vi "RFmx_MeasTest_Config.vi"(7 "Meas_Type":string[](array[string])=["ACP"], 8 "error in (no error)":errorcluster, 11 "Instrument Handle in":refnum<k21>="VST") -> (0 "error out":errorcluster, 3 "Instrument Handle out":refnum<k21>="VST")   [LabVIEW 2014]
uses:
  <vilib>/RFmx/RFInstr/mx/RFmxInstr.llb/RFmxInstr Build Signal String.vi
  <vilib>/RFmx/SpecAn/mx/RFmxSpecAn.llb/RFmxSpecAn Select Measurement (Single).vi
panel:
  in  "Reference Level (dBm)":dbl=-15.0 format="%.2f"
  in  "Enable All Traces":bool=TRUE
  in  "IBW (hz)":dbl=3840000.0 format="%.3p"
  in  "Center Freq (Hz)":dbl=1150000000.0 format="%.3p"
  in  "RBW Filter Type":i32(ring)=1 items=["FFT Based", "Gaussian", "Flat", "Synch Tuned - 4", "Synch Tuned - 5"]
  in  "RBW (Hz)":dbl=10000.0 format="%.3p"
  in  "Span (Hz)":dbl=20000000.0 format="%.3p"
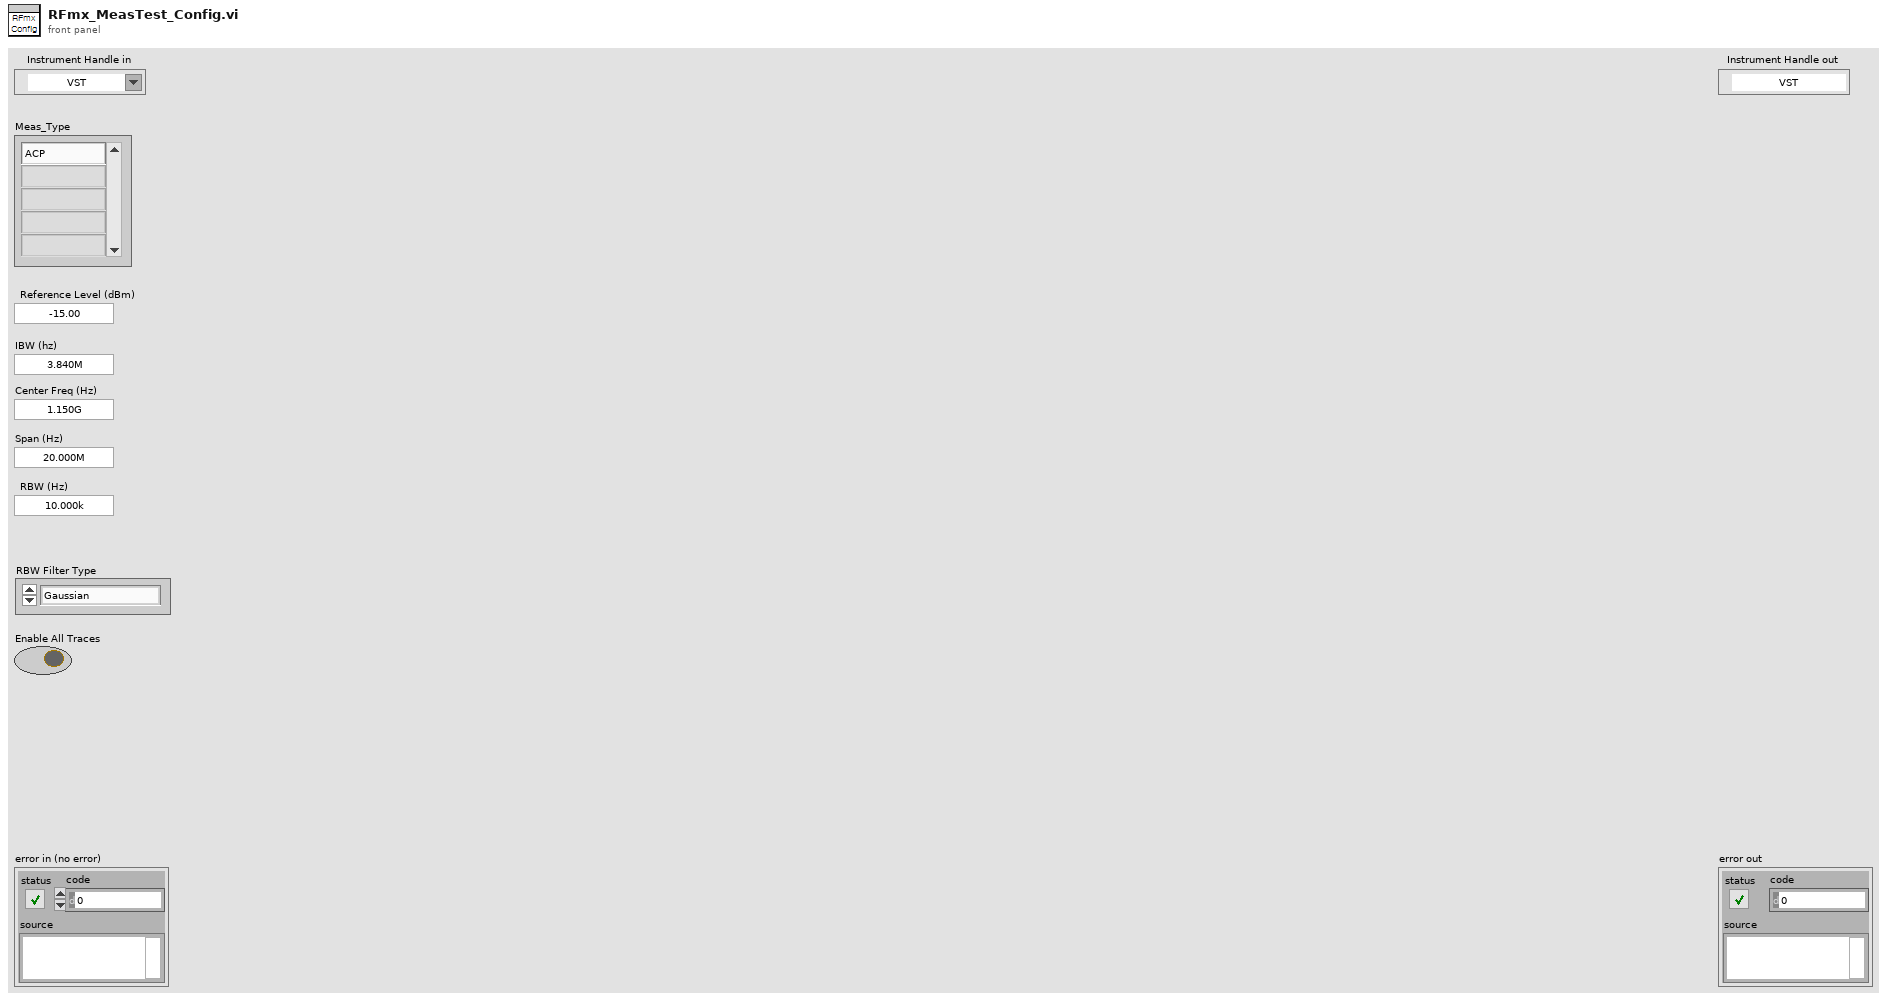
[diagram p1: front panel]
types:
  T1 = enum16{"ACP", "CCDF", "CHP", "FCnt", "Harmonics", "OBW", "SEM", "Spectrum", "Spur", "TXP", "AMPM", "DPD", "IQ"}
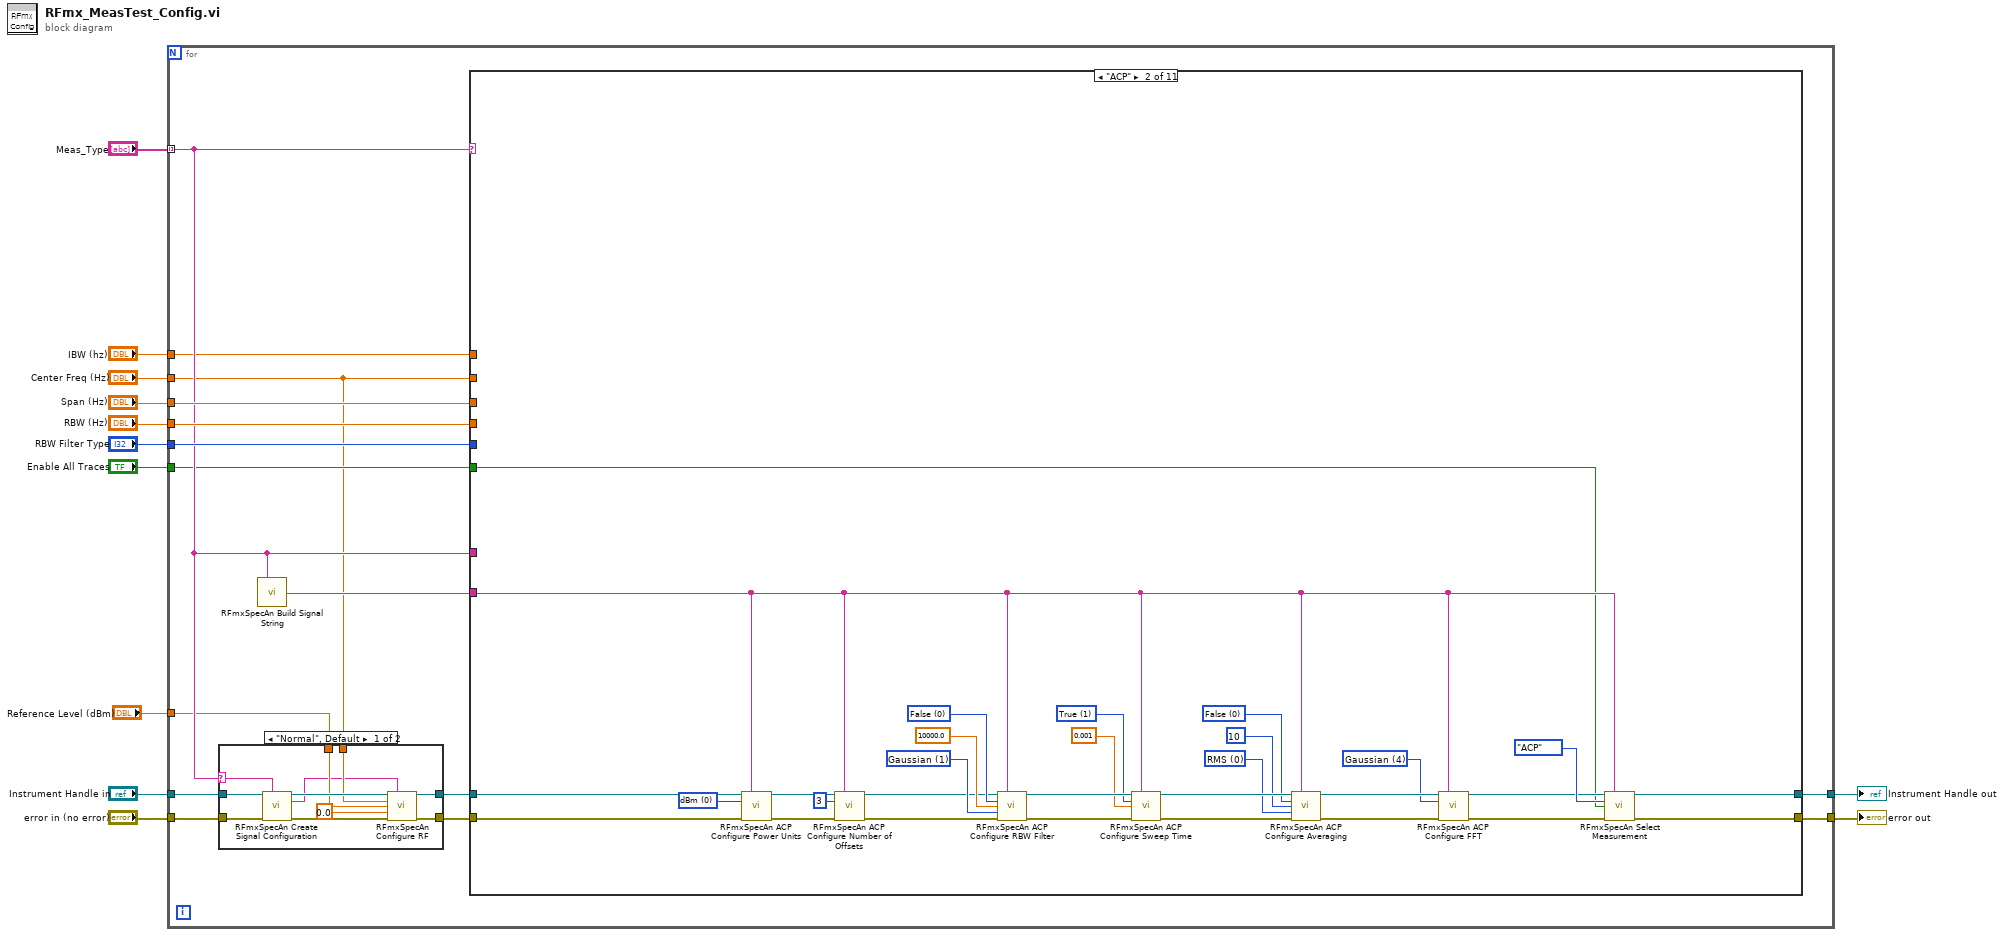
[diagram p0: block diagram]
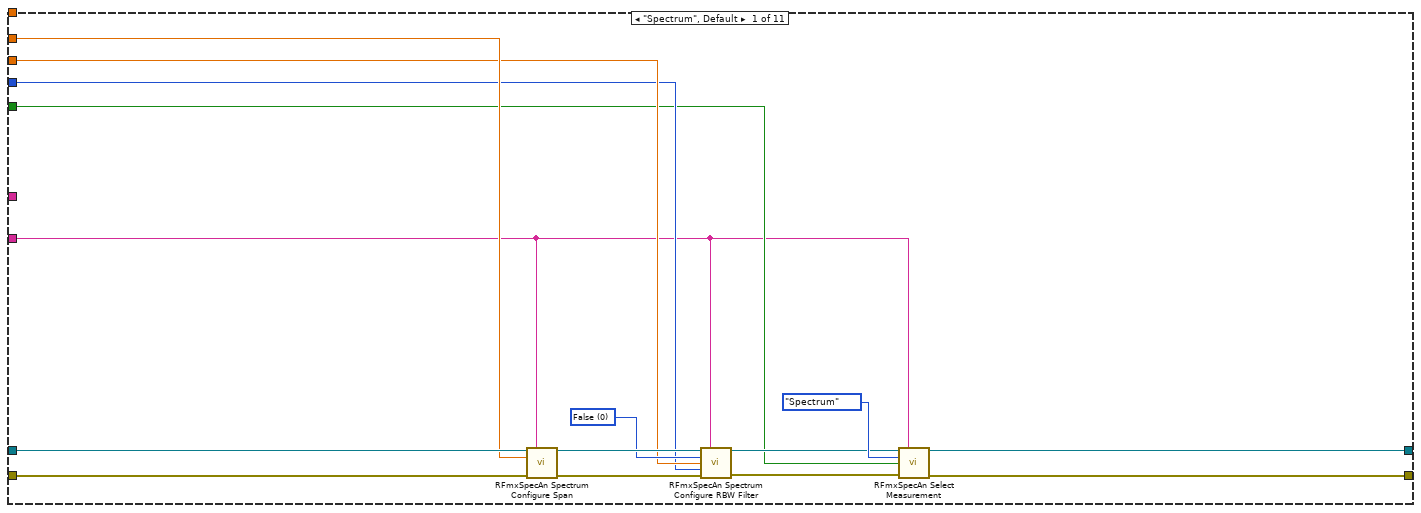
[diagram p3: hidden frame]
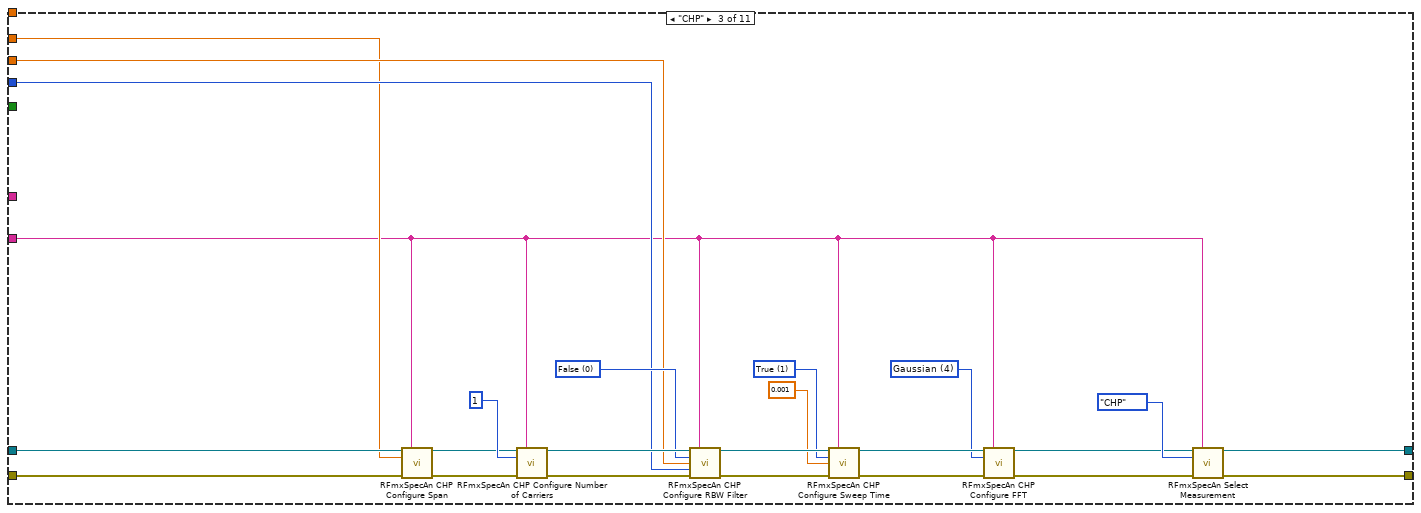
[diagram p4: hidden frame]
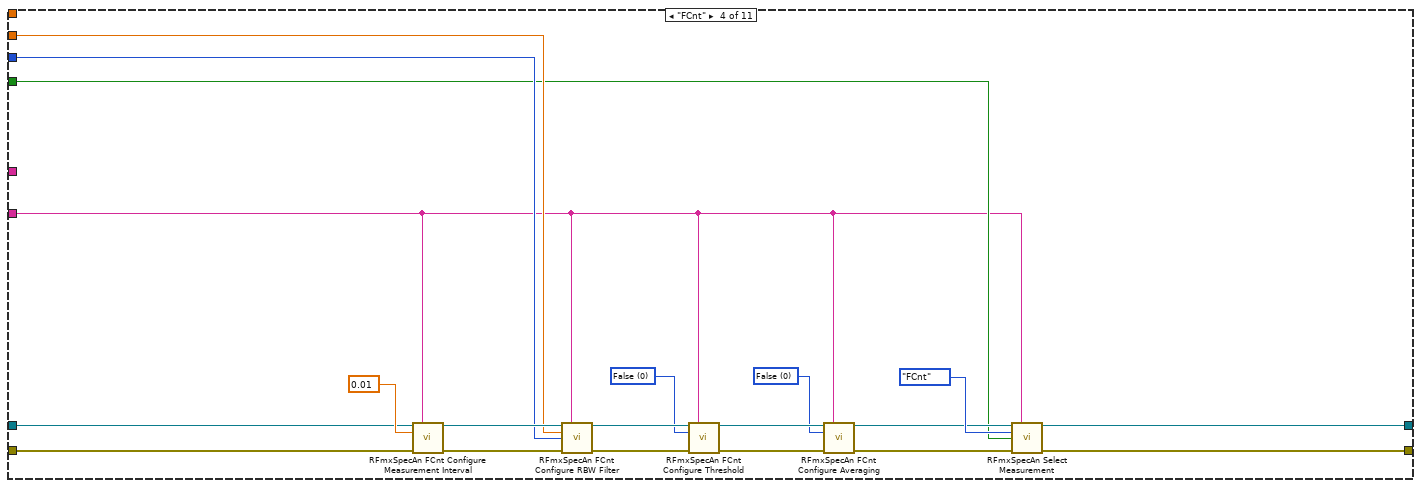
[diagram p5: hidden frame]
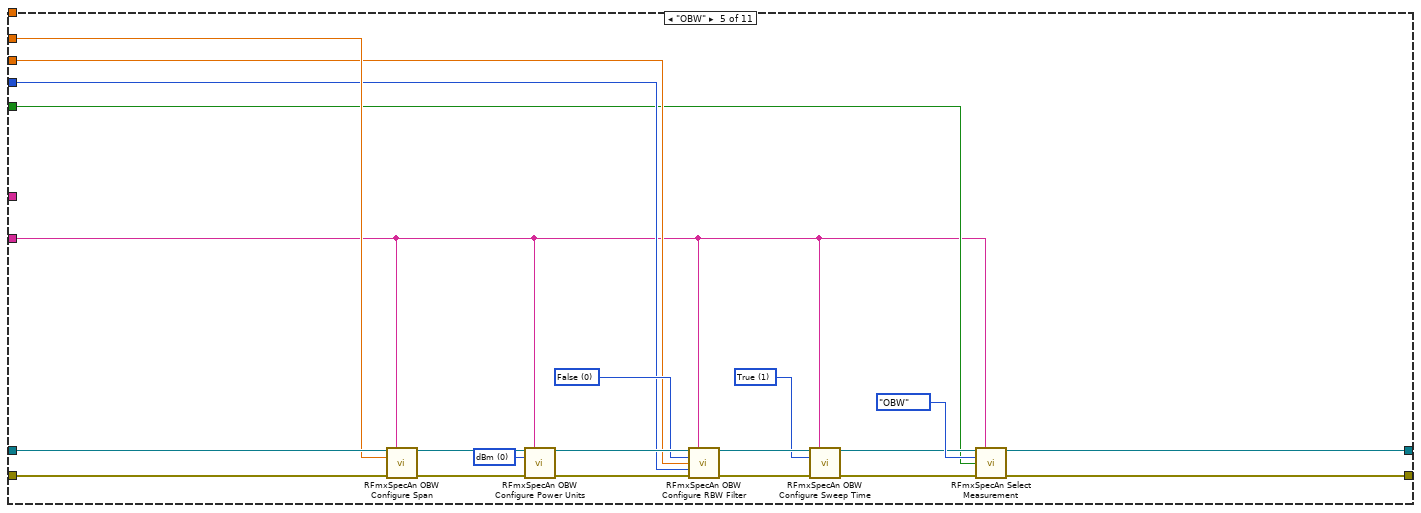
[diagram p6: hidden frame]
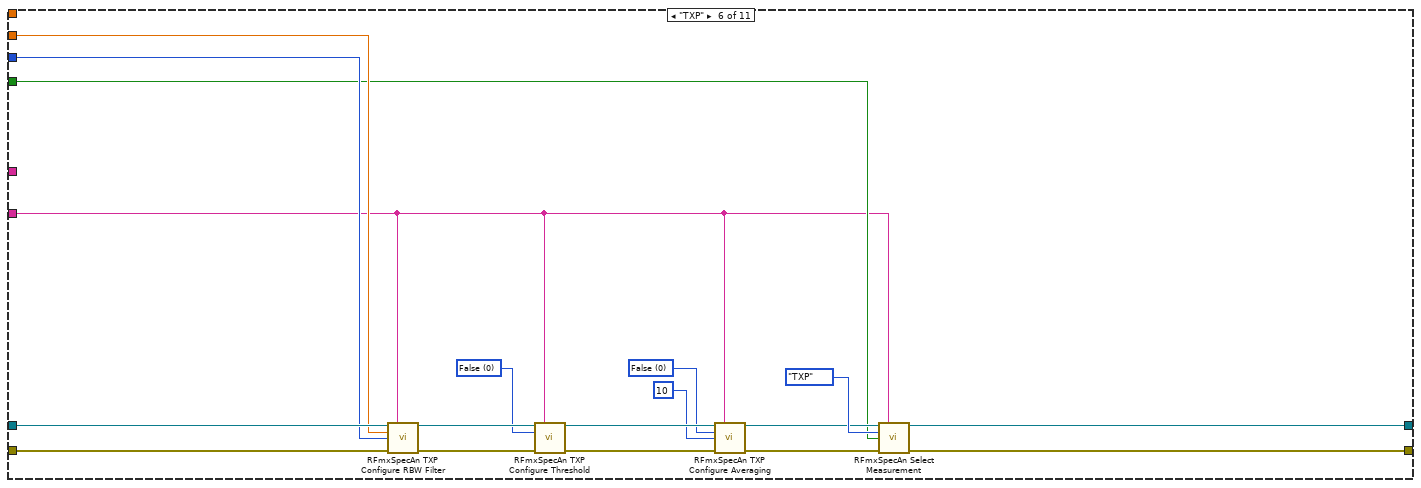
[diagram p7: hidden frame]
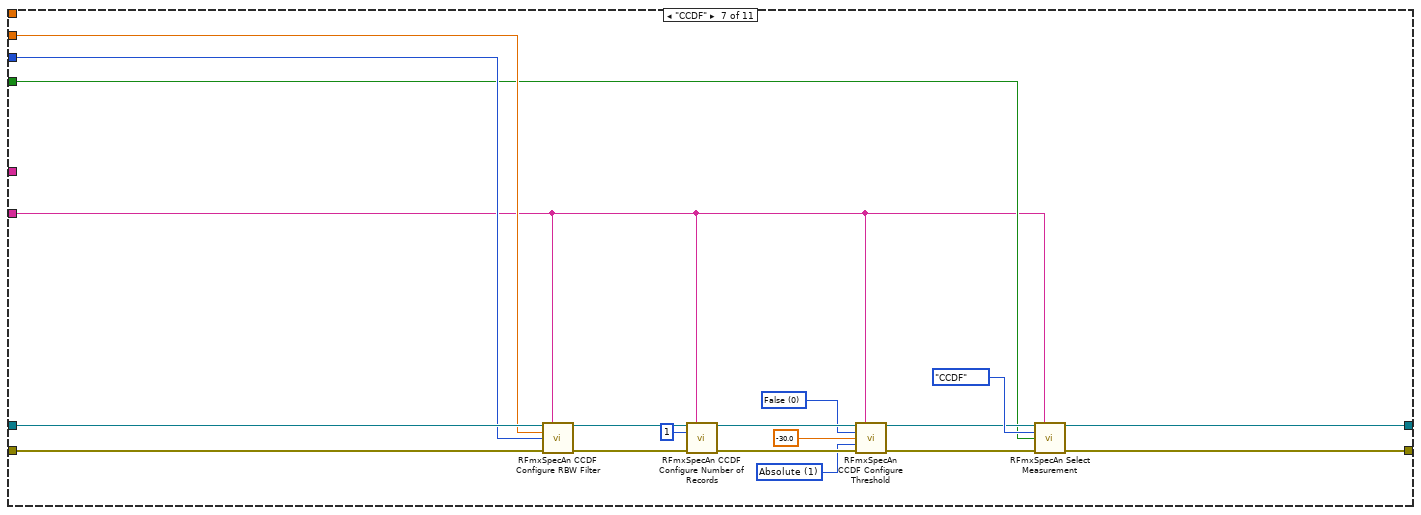
[diagram p8: hidden frame]
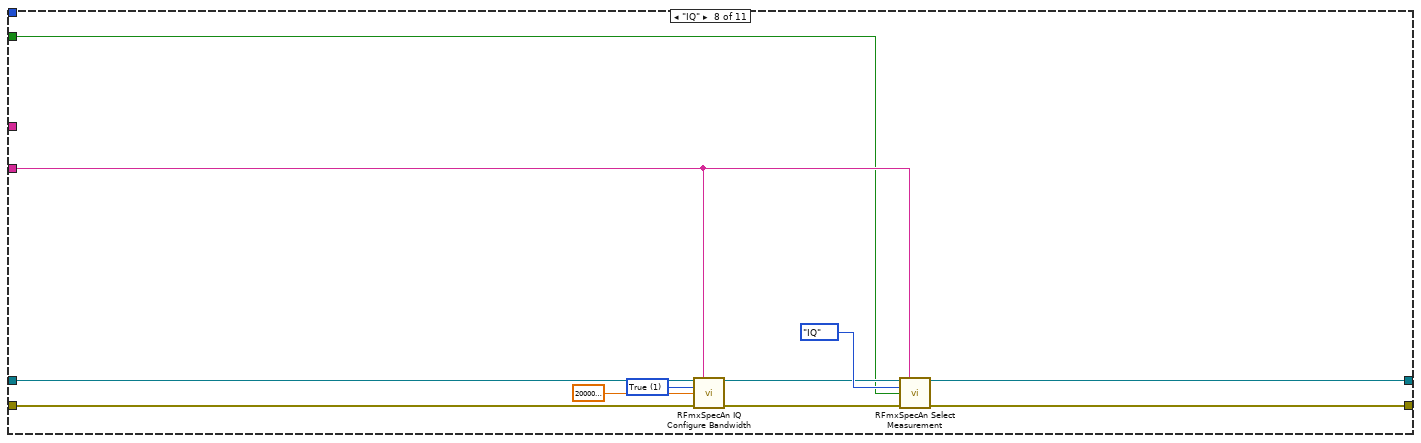
[diagram p9: hidden frame]
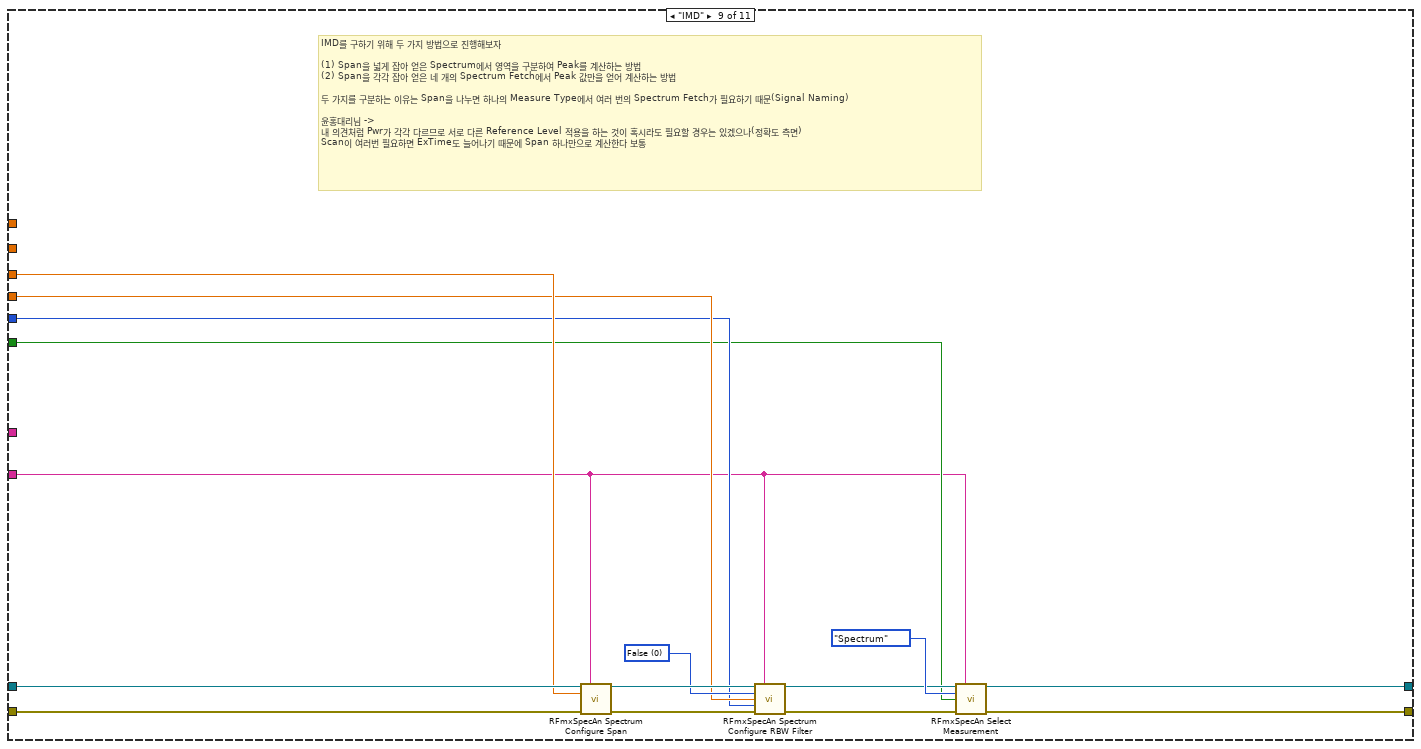
[diagram p10: hidden frame]
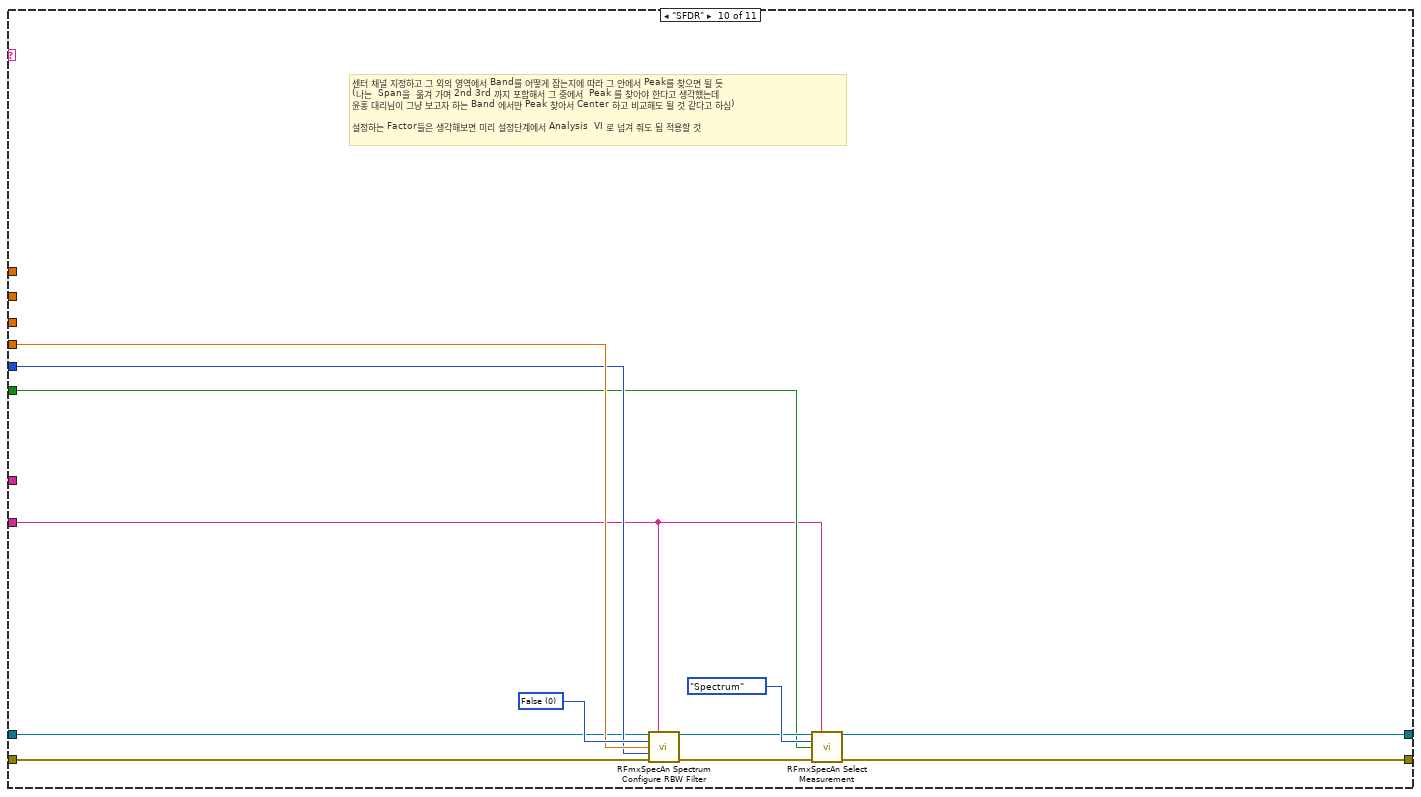
[diagram p11: hidden frame]
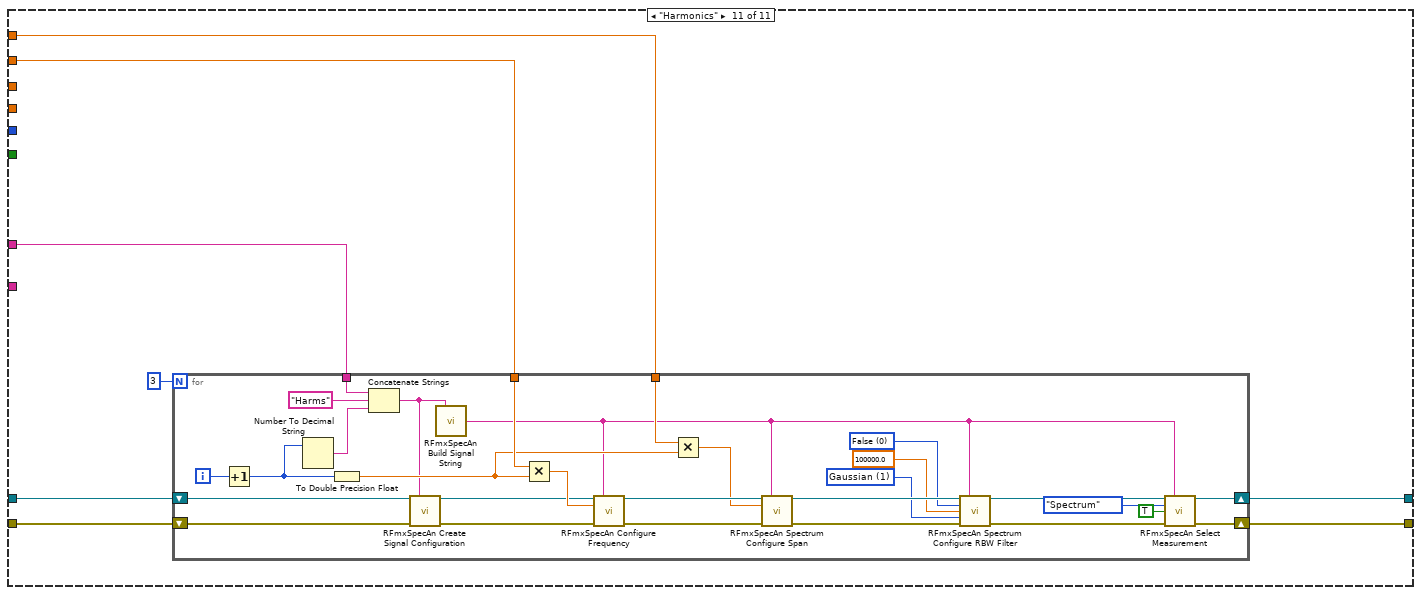
[diagram p12: hidden frame]
diagram:
  n1 = for {
    tunnel: [w27] -> w12
    tunnel: [w26] -> w11
    tunnel: "Meas_Type" -> [w20] mode=indexing
    tunnel: "Instrument Handle in" -> [w22]
    tunnel: "error in (no error)" -> [w21]
    tunnel: "Span (Hz)" -> [w25]
    tunnel: "RBW (Hz)" -> [w24]
    tunnel: "RBW Filter Type" -> [w23]
    tunnel: "Center Freq (Hz)" -> [w15]
    tunnel: "IBW (hz)" -> [w19]
    tunnel: "Enable All Traces" -> [w18]
    tunnel: "Reference Level (dBm)" -> [w16]
    n2 = case shown="\"Normal\", Default" w20 {
      selector: w20 -> [w29 _]
      tunnel: w22 -> [w38 w40]
      tunnel: w21 -> [w37 w39]
      tunnel: [w34 w40] -> w14
      tunnel: [w33 w39] -> w13
      tunnel: w16 -> [w31 _]
      tunnel: w15 -> [w30 _]
      frame "Normal", Default {
        n3 = call <vilib>:"RFmxSpecAn Create Signal Configuration.vi"("Instrument Handle In"=w38, "Signal Name"=w29, "error in (no error)"=w37) -> ("Instrument Handle Out"=w35:refnum<k21>, "Selector String Out"=w28:string, "error out"=w32:errorcluster)  [unwired: 10 in]
        n4 = call <vilib>:"RFmxSpecAn Configure RF.vi"("Instrument Handle In"=w35, "Selector String"=w28, "Center Frequency (Hz)"=w30, "Reference Level (dBm)"=w31, "External Attenuation (dB)"=0.0, "error in (no error)"=w32) -> ("Instrument Handle Out"=w34:refnum<k21>, "error out"=w33:errorcluster)  [unwired: 8 in]
      }
      frame "Harmonics" {
      }
    }
    n5 = call <vilib>:"RFmxSpecAn Build Signal String.vi"("Signal Name"=w20) -> ("Selector String"=w17:string)  [unwired: 14 in]
    n6 = case shown="\"ACP\"" w20 {
      tunnel: w14 -> [w52 w64 w98 w120 w141 w161 w187 w196 w210 w222 w232]
      tunnel: w13 -> [w51 w63 w97 w119 w140 w160 w186 w195 w209 w221 w231]
      tunnel: [w44 w59 w88 w111 w132 w152 w170 w189 w202 w215 w230] -> w26
      tunnel: [w43 w58 w87 w110 w131 w151 w169 w188 w201 w214 w229] -> w27
      tunnel: w25 -> [w50 _ w94 _ w139 _ _ _ w208 _ _]
      tunnel: w24 -> [w49 _ w96 w118 w138 w159 w181 _ w207 w224 _]
      tunnel: w23 -> [w48 _ w95 w117 w137 w158 w180 _ w206 w223 _]
      tunnel: w17 -> [w41 w57 w86 w112 w130 w153 w171 w191 w199 w216 _]
      tunnel: w20 -> [_ _ _ _ _ _ _ _ _ _ w228]
      tunnel: w15 -> [_ _ _ _ _ _ _ _ _ _ w227]
      tunnel: w19 -> [_ _ _ _ _ _ _ _ _ _ w226]
      tunnel: w18 -> [w42 w56 _ w113 w133 w154 w172 w190 w200 w217 _]
      frame "Spectrum", Default {
        w53 = 0 items=["False", "True"] ("RBW Auto")
        n7 = call <vilib>:"RFmxSpecAn Spectrum Configure Span.vi"("Instrument Handle In"=w52, "Selector String"=w41, "Span (Hz)"=w50, "error in (no error)"=w51) -> ("Instrument Handle Out"=w55:refnum<k21>, "error out"=w54:errorcluster)  [unwired: 10 in]
        n8 = call <vilib>:"RFmxSpecAn Spectrum Configure RBW Filter.vi"("Instrument Handle In"=w55, "Selector String"=w41, "RBW Auto"=w53, "RBW (Hz)"=w49, "RBW Filter Type"=w48, "error in (no error)"=w54) -> ("Instrument Handle Out"=w46:refnum<k21>, "error out"=w45:errorcluster)  [unwired: 8 in]
        n9 = call-poly <vilib>:"RFmxSpecAn Select Measurement.vi"("Instrument Handle In"=w46, "Selector String"=w41, "Measurement"=T1."Spectrum", "Enable All Traces"=w42, "error in (no error)"=w45) -> ("Instrument Handle Out"=w44:refnum<k21>, "error out"=w43:errorcluster)  [unwired: 9 in]
      }
      frame "ACP" {
        w71 = 1 items=["False", "True"] ("Sweep Time Auto")
        w72 = 0 items=["RMS", "Log", "Scalar", "Max", "Min", "Vector"] ("Averaging Type")
        w74 = 0 items=["False", "True"] ("Averaging Enabled")
        w75 = 4 items=["None", "Flat Top", "Hanning", "Hamming", "Gaussian", "Blackman", "Blackman-Harris", "Kaiser-Bessel"] ("FFT Window")
        w82 = 1 items=["FFT Based", "Gaussian", "Flat", "Synch Tuned - 4", "Synch Tuned - 5"] ("RBW Filter Type")
        w84 = 0 items=["False", "True"] ("RBW Auto")
        w85 = 0 items=["dBm", "dBm/Hz"] ("Power Units")
        n10 = call <vilib>:"RFmxSpecAn ACP Configure Power Units.vi"("Instrument Handle In"=w64, "Selector String"=w57, "Power Units"=w85, "error in (no error)"=w63) -> ("Instrument Handle Out"=w69:refnum<k21>, "error out"=w68:errorcluster)  [unwired: 10 in]
        n11 = call <vilib>:"RFmxSpecAn ACP Configure Number of Offsets.vi"("Instrument Handle In"=w69, "Selector String"=w57, "Number of Offsets"=3, "error in (no error)"=w68) -> ("Instrument Handle Out"=w67:refnum<k21>, "error out"=w66:errorcluster)  [unwired: 10 in]
        n12 = call <vilib>:"RFmxSpecAn ACP Configure RBW Filter.vi"("Instrument Handle In"=w67, "Selector String"=w57, "RBW Auto"=w84, "RBW (Hz)"=10000.0, "RBW Filter Type"=w82, "error in (no error)"=w66) -> ("Instrument Handle Out"=w81:refnum<k21>, "error out"=w80:errorcluster)  [unwired: 8 in]
        n13 = call <vilib>:"RFmxSpecAn ACP Configure Sweep Time.vi"("Instrument Handle In"=w81, "Selector String"=w57, "Sweep Time Auto"=w71, "Sweep Time Interval (s)"=0.001, "error in (no error)"=w80) -> ("Instrument Handle Out"=w79:refnum<k21>, "error out"=w78:errorcluster)  [unwired: 9 in]
        n14 = call <vilib>:"RFmxSpecAn ACP Configure Averaging.vi"("Instrument Handle In"=w79, "Selector String"=w57, "Averaging Enabled"=w74, "Averaging Count"=10, "Averaging Type"=w72, "error in (no error)"=w78) -> ("Instrument Handle Out"=w77:refnum<k21>, "error out"=w76:errorcluster)  [unwired: 8 in]
        n15 = call <vilib>:"RFmxSpecAn ACP Configure FFT.vi"("Instrument Handle In"=w77, "Selector String"=w57, "FFT Window"=w75, "error in (no error)"=w76) -> ("Instrument Handle Out"=w61:refnum<k21>, "error out"=w60:errorcluster)  [unwired: 10 in]
        n16 = call-poly <vilib>:"RFmxSpecAn Select Measurement.vi"("Instrument Handle In"=w61, "Selector String"=w57, "Measurement"=T1."ACP", "Enable All Traces"=w56, "error in (no error)"=w60) -> ("Instrument Handle Out"=w59:refnum<k21>, "error out"=w58:errorcluster)  [unwired: 9 in]
      }
      frame "CHP" {
        w99 = 4 items=["None", "Flat Top", "Hanning", "Hamming", "Gaussian", "Blackman", "Blackman-Harris", "Kaiser-Bessel"] ("FFT Window")
        w103 = 1 items=["False", "True"] ("Sweep Time Auto")
        w106 = 0 items=["False", "True"] ("RBW Auto")
        n17 = call <vilib>:"RFmxSpecAn CHP Configure Span.vi"("Instrument Handle In"=w98, "Selector String"=w86, "Span (Hz)"=w94, "error in (no error)"=w97) -> ("Instrument Handle Out"=w93:refnum<k21>, "error out"=w92:errorcluster)  [unwired: 10 in]
        n18 = call <vilib>:"RFmxSpecAn CHP Configure Number of Carriers.vi"("Instrument Handle In"=w93, "Selector String"=w86, "Number of Carriers"=1, "error in (no error)"=w92) -> ("Instrument Handle Out"=w108:refnum<k21>, "error out"=w107:errorcluster)  [unwired: 10 in]
        n19 = call <vilib>:"RFmxSpecAn CHP Configure RBW Filter.vi"("Instrument Handle In"=w108, "Selector String"=w86, "RBW Auto"=w106, "RBW (Hz)"=w96, "RBW Filter Type"=w95, "error in (no error)"=w107) -> ("Instrument Handle Out"=w105:refnum<k21>, "error out"=w104:errorcluster)  [unwired: 8 in]
        n20 = call <vilib>:"RFmxSpecAn CHP Configure Sweep Time.vi"("Instrument Handle In"=w105, "Selector String"=w86, "Sweep Time Auto"=w103, "Sweep Time Interval (s)"=0.001, "error in (no error)"=w104) -> ("Instrument Handle Out"=w101:refnum<k21>, "error out"=w100:errorcluster)  [unwired: 9 in]
        n21 = call <vilib>:"RFmxSpecAn CHP Configure FFT.vi"("Instrument Handle In"=w101, "Selector String"=w86, "FFT Window"=w99, "error in (no error)"=w100) -> ("Instrument Handle Out"=w90:refnum<k21>, "error out"=w89:errorcluster)  [unwired: 10 in]
        n22 = call-poly <vilib>:"RFmxSpecAn Select Measurement.vi"("Instrument Handle In"=w90, "Selector String"=w86, "Measurement"=T1."CHP", "error in (no error)"=w89) -> ("Instrument Handle Out"=w88:refnum<k21>, "error out"=w87:errorcluster)  [unwired: 10 in]
      }
      frame "FCnt" {
        w122 = 0 items=["False", "True"] ("Averaging Enabled")
        w124 = 0 items=["False", "True"] ("Threshold Enabled")
        n23 = call <vilib>:"RFmxSpecAn FCnt Configure Measurement Interval.vi"("Instrument Handle In"=w120, "Selector String"=w112, "Measurement Interval (s)"=0.01, "error in (no error)"=w119) -> ("Instrument Handle Out"=w128:refnum<k21>, "error out"=w127:errorcluster)  [unwired: 10 in]
        n24 = call <vilib>:"RFmxSpecAn FCnt Configure RBW Filter.vi"("Instrument Handle In"=w128, "Selector String"=w112, "RBW (Hz)"=w118, "RBW Filter Type"=w117, "error in (no error)"=w127) -> ("Instrument Handle Out"=w126:refnum<k21>, "error out"=w125:errorcluster)  [unwired: 9 in]
        n25 = call <vilib>:"RFmxSpecAn FCnt Configure Threshold.vi"("Instrument Handle In"=w126, "Selector String"=w112, "Threshold Enabled"=w124, "error in (no error)"=w125) -> ("Instrument Handle Out"=w123:refnum<k21>, "error out"=w121:errorcluster)  [unwired: 10 in]
        n26 = call <vilib>:"RFmxSpecAn FCnt Configure Averaging.vi"("Instrument Handle In"=w123, "Selector String"=w112, "Averaging Enabled"=w122, "error in (no error)"=w121) -> ("Instrument Handle Out"=w115:refnum<k21>, "error out"=w114:errorcluster)  [unwired: 10 in]
        n27 = call-poly <vilib>:"RFmxSpecAn Select Measurement.vi"("Instrument Handle In"=w115, "Selector String"=w112, "Measurement"=T1."FCnt", "Enable All Traces"=w113, "error in (no error)"=w114) -> ("Instrument Handle Out"=w111:refnum<k21>, "error out"=w110:errorcluster)  [unwired: 9 in]
      }
      frame "OBW" {
        w142 = 1 items=["False", "True"] ("Sweep Time Auto")
        w145 = 0 items=["False", "True"] ("RBW Auto")
        w148 = 0 items=["dBm", "dBm/Hz"] ("Power Units")
        n28 = call <vilib>:"RFmxSpecAn OBW Configure Span.vi"("Instrument Handle In"=w141, "Selector String"=w130, "Span (Hz)"=w139, "error in (no error)"=w140) -> ("Instrument Handle Out"=w150:refnum<k21>, "error out"=w149:errorcluster)  [unwired: 10 in]
        n29 = call <vilib>:"RFmxSpecAn OBW Configure Power Units.vi"("Instrument Handle In"=w150, "Selector String"=w130, "Power Units"=w148, "error in (no error)"=w149) -> ("Instrument Handle Out"=w147:refnum<k21>, "error out"=w146:errorcluster)  [unwired: 10 in]
        n30 = call <vilib>:"RFmxSpecAn OBW Configure RBW Filter.vi"("Instrument Handle In"=w147, "Selector String"=w130, "RBW Auto"=w145, "RBW (Hz)"=w138, "RBW Filter Type"=w137, "error in (no error)"=w146) -> ("Instrument Handle Out"=w144:refnum<k21>, "error out"=w143:errorcluster)  [unwired: 8 in]
        n31 = call <vilib>:"RFmxSpecAn OBW Configure Sweep Time.vi"("Instrument Handle In"=w144, "Selector String"=w130, "Sweep Time Auto"=w142, "error in (no error)"=w143) -> ("Instrument Handle Out"=w135:refnum<k21>, "error out"=w134:errorcluster)  [unwired: 10 in]
        n32 = call-poly <vilib>:"RFmxSpecAn Select Measurement.vi"("Instrument Handle In"=w135, "Selector String"=w130, "Measurement"=T1."OBW", "Enable All Traces"=w133, "error in (no error)"=w134) -> ("Instrument Handle Out"=w132:refnum<k21>, "error out"=w131:errorcluster)  [unwired: 9 in]
      }
      frame "TXP" {
        w163 = 0 items=["False", "True"] ("Averaging Enabled")
        w167 = 0 items=["False", "True"] ("Threshold Enabled")
        n33 = call <vilib>:"RFmxSpecAn TXP Configure RBW Filter.vi"("Instrument Handle In"=w161, "Selector String"=w153, "RBW (Hz)"=w159, "RBW Filter Type"=w158, "error in (no error)"=w160) -> ("Instrument Handle Out"=w168:refnum<k21>, "error out"=w166:errorcluster)  [unwired: 9 in]
        n34 = call <vilib>:"RFmxSpecAn TXP Configure Threshold.vi"("Instrument Handle In"=w168, "Selector String"=w153, "Threshold Enabled"=w167, "error in (no error)"=w166) -> ("Instrument Handle Out"=w165:refnum<k21>, "error out"=w164:errorcluster)  [unwired: 10 in]
        n35 = call <vilib>:"RFmxSpecAn TXP Configure Averaging.vi"("Instrument Handle In"=w165, "Selector String"=w153, "Averaging Enabled"=w163, "Averaging Count"=10, "error in (no error)"=w164) -> ("Instrument Handle Out"=w156:refnum<k21>, "error out"=w155:errorcluster)  [unwired: 9 in]
        n36 = call-poly <vilib>:"RFmxSpecAn Select Measurement.vi"("Instrument Handle In"=w156, "Selector String"=w153, "Measurement"=T1."TXP", "Enable All Traces"=w154, "error in (no error)"=w155) -> ("Instrument Handle Out"=w152:refnum<k21>, "error out"=w151:errorcluster)  [unwired: 9 in]
      }
      frame "CCDF" {
        w176 = 1 items=["Relative", "Absolute"] ("Threshold Type")
        w178 = 0 items=["False", "True"] ("Threshold Enabled")
        n37 = call <vilib>:"RFmxSpecAn CCDF Configure RBW Filter.vi"("Instrument Handle In"=w187, "Selector String"=w171, "RBW (Hz)"=w181, "RBW Filter Type"=w180, "error in (no error)"=w186) -> ("Instrument Handle Out"=w185:refnum<k21>, "error out"=w184:errorcluster)  [unwired: 9 in]
        n38 = call <vilib>:"RFmxSpecAn CCDF Configure Number of Records.vi"("Instrument Handle In"=w185, "Selector String"=w171, "Number of Records"=1, "error in (no error)"=w184) -> ("Instrument Handle Out"=w183:refnum<k21>, "error out"=w182:errorcluster)  [unwired: 10 in]
        n39 = call <vilib>:"RFmxSpecAn CCDF Configure Threshold.vi"("Instrument Handle In"=w183, "Selector String"=w171, "Threshold Enabled"=w178, "Threshold Level (dB or dBm)"=-30.0, "Threshold Type"=w176, "error in (no error)"=w182) -> ("Instrument Handle Out"=w174:refnum<k21>, "error out"=w173:errorcluster)  [unwired: 8 in]
        n40 = call-poly <vilib>:"RFmxSpecAn Select Measurement.vi"("Instrument Handle In"=w174, "Selector String"=w171, "Measurement"=T1."CCDF", "Enable All Traces"=w172, "error in (no error)"=w173) -> ("Instrument Handle Out"=w170:refnum<k21>, "error out"=w169:errorcluster)  [unwired: 9 in]
      }
      frame "IQ" {
        w197 = 1 items=["False", "True"] ("Bandwidth Auto")
        n41 = call <vilib>:"RFmxSpecAn IQ Configure Bandwidth.vi"("Instrument Handle In"=w196, "Selector String"=w191, "Bandwidth Auto"=w197, "Bandwidth (Hz)"=20000000.0, "error in (no error)"=w195) -> ("Instrument Handle Out"=w193:refnum<k21>, "error out"=w192:errorcluster)  [unwired: 9 in]
        n42 = call-poly <vilib>:"RFmxSpecAn Select Measurement.vi"("Instrument Handle In"=w193, "Selector String"=w191, "Measurement"=T1."IQ", "Enable All Traces"=w190, "error in (no error)"=w192) -> ("Instrument Handle Out"=w189:refnum<k21>, "error out"=w188:errorcluster)  [unwired: 9 in]
      }
      frame "IMD" {
        w211 = 0 items=["False", "True"] ("RBW Auto")
        # "IMD를 구하기 위해 두 가지 방법으로 진행해보자\n\n(1) Span을 넓게 잡아 얻은 Spectrum에서 영역을 구분하여 Peak를 계산하는 방법\n(2) Span을 각각 잡아 얻은 네 개의 Spectrum Fetch에서 Peak 값만을 얻어 계산하는 방법\n\n두 가지를 구분하는 이유는 Span을 나누면 하나의 Measure Type에서 여러 번의 Spectrum Fetch가 필요하기 때문(Signal Naming)\n\n윤홍대리님 -> \n내 의견처럼 Pwr가 각각 다르므로 서로 다른 Reference Level 적용을 하는 것이 혹시라도 필요할 경우는 있겠으나(정확도 측면)\nScan이 여러번 필요하면 ExTime도 늘어나기 때문에 Span 하나만으로 계산한다 보통"
        n43 = call <vilib>:"RFmxSpecAn Spectrum Configure Span.vi"("Instrument Handle In"=w210, "Selector String"=w199, "Span (Hz)"=w208, "error in (no error)"=w209) -> ("Instrument Handle Out"=w213:refnum<k21>, "error out"=w212:errorcluster)  [unwired: 10 in]
        n44 = call <vilib>:"RFmxSpecAn Spectrum Configure RBW Filter.vi"("Instrument Handle In"=w213, "Selector String"=w199, "RBW Auto"=w211, "RBW (Hz)"=w207, "RBW Filter Type"=w206, "error in (no error)"=w212) -> ("Instrument Handle Out"=w204:refnum<k21>, "error out"=w203:errorcluster)  [unwired: 8 in]
        n45 = call-poly <vilib>:"RFmxSpecAn Select Measurement.vi"("Instrument Handle In"=w204, "Selector String"=w199, "Measurement"=T1."Spectrum", "Enable All Traces"=w200, "error in (no error)"=w203) -> ("Instrument Handle Out"=w202:refnum<k21>, "error out"=w201:errorcluster)  [unwired: 9 in]
      }
      frame "SFDR" {
        w225 = 0 items=["False", "True"] ("RBW Auto")
        # "센터 채널 지정하고 그 외의 영역에서 Band를 어떻게 잡는지에 따라 그 안에서 Peak를 찾으면 될 듯\n(나는  Span을  옮겨 가며 2nd 3rd 까지 포함해서 그 중에서  Peak 를 찾아야 한다고 생각했는데\n윤홍 대리님이 그냥 보고자 하는 Band 에서만 Peak 찾아서 Center 하고 비교해도 될 것 같다고 하심)\n\n설정하는 Factor들은 생각해보면 미리 설정단계에서 Analysis  VI 로 넘겨 줘도 됨 적용할 것"
        n46 = call <vilib>:"RFmxSpecAn Spectrum Configure RBW Filter.vi"("Instrument Handle In"=w222, "Selector String"=w216, "RBW Auto"=w225, "RBW (Hz)"=w224, "RBW Filter Type"=w223, "error in (no error)"=w221) -> ("Instrument Handle Out"=w219:refnum<k21>, "error out"=w218:errorcluster)  [unwired: 8 in]
        n47 = call-poly <vilib>:"RFmxSpecAn Select Measurement.vi"("Instrument Handle In"=w219, "Selector String"=w216, "Measurement"=T1."Spectrum", "Enable All Traces"=w217, "error in (no error)"=w218) -> ("Instrument Handle Out"=w215:refnum<k21>, "error out"=w214:errorcluster)  [unwired: 9 in]
      }
      frame "Harmonics" {
        n48 = for {
          N: 3 -> [_]
          shift-right: [w240] -> w230
          shift-left: w232 -> [w248]
          shift-right: [w239] -> w229
          shift-left: w231 -> [w247]
          tunnel: w227 -> [w257]
          tunnel: w226 -> [w256]
          tunnel: w228 -> [w237]
          i -> [w235]
          w251 = 1 items=["FFT Based", "Gaussian", "Flat", "Synch Tuned - 4", "Synch Tuned - 5"] ("RBW Filter Type")
          w253 = 0 items=["False", "True"] ("RBW Auto")
          n49 = Increment(x=w235) -> (x+1=w234:i32)
          n50 = Number To Decimal String(number=w234) -> (decimal integer string=w249:string)  [unwired: 1 in]
          n51 = To Double Precision Float(number=w234) -> (double precision float=w255:dbl)
          n52 = Concatenate Strings(w237, "Harms", w249) -> (w246:string)
          n53 = call <vilib>:"RFmxSpecAn Create Signal Configuration.vi"("Instrument Handle In"=w248, "Signal Name"=w246, "error in (no error)"=w247) -> ("Instrument Handle Out"=w245:refnum<k21>, "error out"=w244:errorcluster)  [unwired: 10 in, 1 out]
          n54 = call <vilib>:"RFmxSpecAn Build Signal String.vi"("Signal Name"=w246) -> ("Selector String"=w238:string)  [unwired: 14 in]
          n55 = Multiply(x=w257, y=w255) -> (x*y=w258:dbl)
          n56 = call <vilib>:"RFmxSpecAn Configure Frequency.vi"("Instrument Handle In"=w245, "Selector String"=w238, "Center Frequency (Hz)"=w258, "error in (no error)"=w244) -> ("Instrument Handle Out"=w262:refnum<k21>, "error out"=w261:errorcluster)  [unwired: 10 in]
          n57 = Multiply(x=w256, y=w255) -> (x*y=w254:dbl)
          n58 = call <vilib>:"RFmxSpecAn Spectrum Configure Span.vi"("Instrument Handle In"=w262, "Selector String"=w238, "Span (Hz)"=w254, "error in (no error)"=w261) -> ("Instrument Handle Out"=w260:refnum<k21>, "error out"=w259:errorcluster)  [unwired: 10 in]
          n59 = call <vilib>:"RFmxSpecAn Spectrum Configure RBW Filter.vi"("Instrument Handle In"=w260, "Selector String"=w238, "RBW Auto"=w253, "RBW (Hz)"=100000.0, "RBW Filter Type"=w251, "error in (no error)"=w259) -> ("Instrument Handle Out"=w243:refnum<k21>, "error out"=w242:errorcluster)  [unwired: 8 in]
          n60 = call-poly <vilib>:"RFmxSpecAn Select Measurement.vi"("Instrument Handle In"=w243, "Selector String"=w238, "Measurement"=T1."Spectrum", "Enable All Traces"=TRUE, "error in (no error)"=w242) -> ("Instrument Handle Out"=w240:refnum<k21>, "error out"=w239:errorcluster)  [unwired: 9 in]
        }
      }
    }
  }
  "Instrument Handle out" <- w11
  "error out" <- w12
